vi "Read.vi"(7 "timeout (100ms)":i32=100, 8 "error in (no error)":errorcluster, 9 "Interlock in":bool, 11 "Interlock Bool in":refnum<class "Interlock Range.lvclass">) -> (0 "error out":errorcluster, 1 "Interlock":bool, 2 "Data out":variant, 3 "Interlock Bool out":refnum<class "Interlock Range.lvclass">, 4 "IL Action":refnum<class "IL Action.lvclass">[](array[class]))   [LabVIEW 2015, in "Interlocks.lvlib" / "Interlock Range.lvclass"]
uses:
  Interlock Range.lvclass
  IL Action/IL Action.lvclass
  Interlock Range.lvclass/Interlock Range.ctl
  Interlock/State Enum.ctl
  Interlock/Interlock.lvclass/Interlock.ctl
  Interlock/Interlock.lvclass
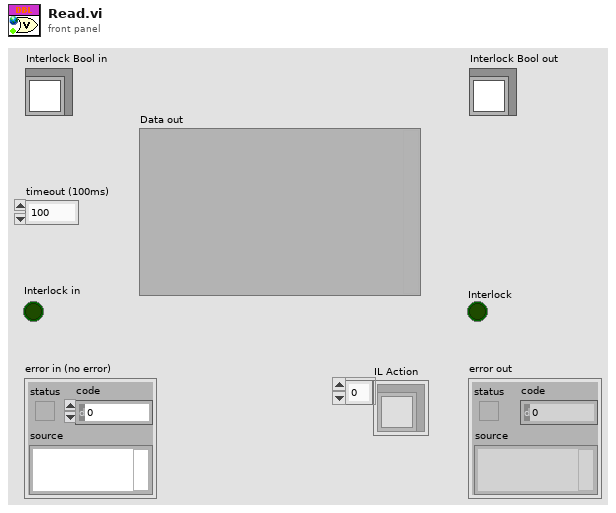
[diagram p1: front panel]
types:
  T1 = typedef "Interlocks.lvlib/Interlock.lvclass/State Enum.ctl" = enum16{"Ok", "Interlock", "Out of Range", "Is ON", "Is OFF", "Error", "Denied", "Not Allowed", "Sample Allow", "Sample Deny"}
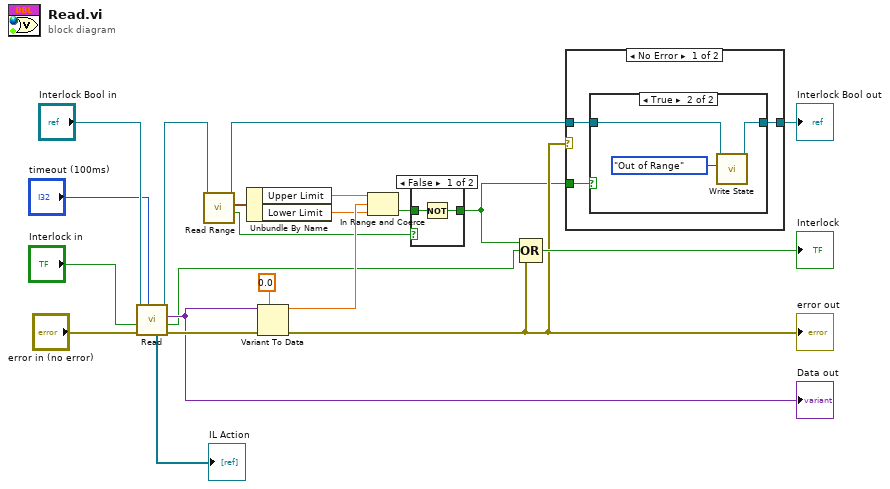
[diagram p0: block diagram]
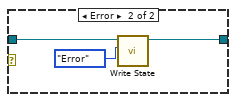
[diagram p4: hidden frame]
diagram:
  n1 = call-parent "Read.vi"("timeout (100ms)"="timeout (100ms)", "error in (no error)"="error in (no error)", 9:"Interlock in"="Interlock in", 11:"Interlock in"="Interlock Bool in") -> ("error out"=w18:errorcluster, 1:"Interlock out"=w8:bool, "Data out"=w16:variant, 3:"Interlock out"=w19:refnum<class "Interlock Range.lvclass">, "IL Action"=→"IL Action":refnum<class "IL Action.lvclass">[])  [unwired: 3 in]
  "Data out" <- w16
  n2 = call "Read Range.vi"("Interlock Bool in"=w19) -> ("Exclude Range"=w1:bool, "Range"=w13:cluster{"Upper Limit":dbl, "Lower Limit":dbl}, "Interlock Bool out"=w6:refnum<class "Interlock Range.lvclass">)  [unwired: 8 in]
  n3 = Unbundle By Name(w13) -> ("Upper Limit"=w12:dbl, "Lower Limit"=w10:dbl)
  n4 = Variant To Data(error in=w18, type=0.0, Variant=w16) -> (data=w11:dbl, error out=w5:errorcluster)
  "error out" <- w5
  n5 = In Range and Coerce(upper limit=w12, x=w11, lower limit=w10) -> (In Range?=w9:bool)  [unwired: 1 out]
  n6 = case shown="False" w1 {
    tunnel: w9 -> [w23 w24]
    tunnel: [w22 w24] -> w2
    frame False {
      n7 = Not(x=w23) -> (.not. x?=w22:bool)
    }
    frame True {
    }
  }
  n8 = Compound Arithmetic op=OR(w2, w8, w5) -> (→"Interlock":bool)
  n9 = case shown="No Error" w5 {
    tunnel: [w26 w34] -> w7
    tunnel: w6 -> [w27 w33]
    tunnel: w2 -> [w25 _]
    frame No Error {
      n10 = case shown="True" w25 {
        tunnel: w27 -> [w28 w31]
        tunnel: [w28 w30] -> w26
        frame False {
        }
        frame True {
          n11 = call "Write State.vi"("State"=State_Enum."Out of Range", "Interlock in"=w31) -> ("Interlock out"=w30:refnum<class "Interlock Range.lvclass">)  [unwired: 9 in]
        }
      }
    }
    frame Error {
      n12 = call "Write State.vi"("State"=State_Enum."Error" ("t"), "Interlock in"=w33) -> ("Interlock out"=w34:refnum<class "Interlock Range.lvclass">)  [unwired: 9 in]
    }
  }
  "Interlock Bool out" <- w7
